vi "configure.vi"(8 "error in (no error)":errorcluster, 9 "Value":i32, 10 "ILC":refnum<class "ILC.lvclass">, 11 "ConfigureILCDOStrategy in":refnum<class "ConfigureILCDOStrategy.lvclass">) -> (0 "error out":errorcluster, 3 "ConfigureILCDOStrategy out":refnum<class "ConfigureILCDOStrategy.lvclass">)   [LabVIEW 2015, in "ConfigureILCDOStrategy.lvclass"]
uses:
  ConfigureILCDOStrategy.lvclass
  <userlib>/Common/ilc/ILC/ILC.lvclass
  ConfigureILCDOStrategy.lvclass/ConfigureILCDOStrategy.ctl
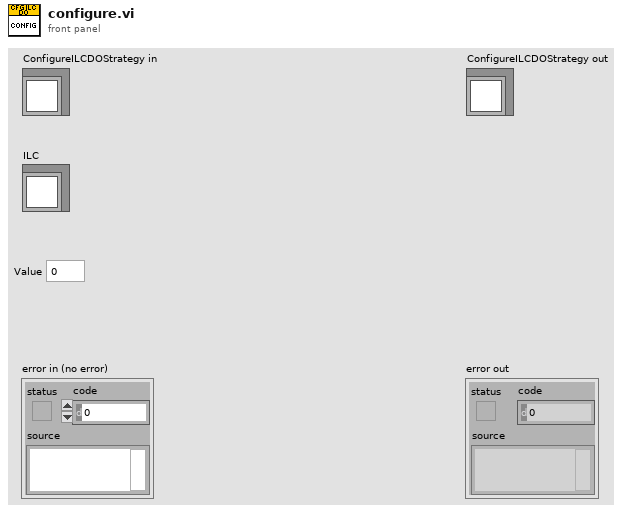
[diagram p1: front panel]
types:
  T1 = typedef "ILCBTTypedefs.lvlib/MUX Settings.ctl" = cluster{"MUX_AO":T2, "MUX_A1":T2, "MUX_A0 DAQ Channel to Write":refnum<k21>, "MUX_A1 DAQ Channel to Write":refnum<k21>}
  T2 = typedef "ILCBTTypedefs.lvlib/Digital Signal Level.ctl" = enum16{"Low", "High"}
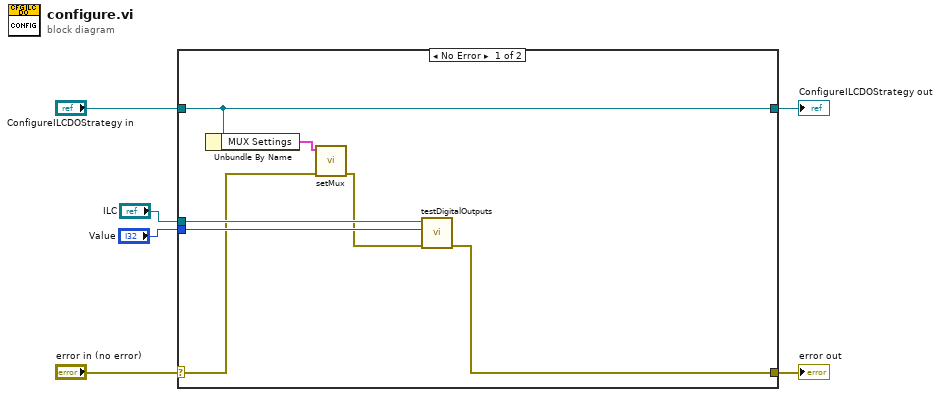
[diagram p0: block diagram]
diagram:
  n1 = case shown="No Error" "error in (no error)" {
    selector: "error in (no error)" -> [w8 w15]
    tunnel: [w7 w15] -> w5
    tunnel: [w13 w14] -> w3
    tunnel: "ConfigureILCDOStrategy in" -> [w13 w14]
    tunnel: "ILC" -> [w11 _]
    tunnel: "Value" -> [w10 _]
    frame No Error {
      n2 = Unbundle By Name(w13) -> ("MUX Settings"=w12:T1)
      n3 = call "setMux.vi"("error in (no error)"=w8, "MUX Settings"=w12) -> ("error out"=w9:errorcluster)  [unwired: 9 in]
      n4 = call <userlib>:"testDigitalOutputs.vi"("error in (no error)"=w9, "Digital Output Value"=w10, "ILC in"=w11) -> ("error out"=w7:errorcluster)  [unwired: 7 in, 1 out]
    }
    frame Error {
    }
  }
  "error out" <- w5
  "ConfigureILCDOStrategy out" <- w3
